vi "Balance Control Design.vi"() -> ()   [LabVIEW 2018]
uses:
  <vilib>/Analysis/baseanly.llb/Real A x B.vi
  <vilib>/Analysis/_algsub.llb/Real Matrix Rank.vi
  <vilib>/addons/Control Design/_Model Construction/Model Creation.llb/Model Creation SubVI/cd_Create State Space Model.vi
  <vilib>/addons/Control Design/_Model Construction/Model Information.llb/Model Information SubVIs/cd_Get Matrices From SS Model.vi
  <vilib>/Analysis/Matrix/Numeric/Subtract/Subtract - RM,RM.vi
  <vilib>/addons/Control Design/_Model Construction/Model Information.llb/Model Information SubVIs/cd_Set Matrices To SS Model.vi
  <vilib>/addons/Control Design/_Dynamic Analysis/Dynamic Analysis.llb/Dynamic Analysis subVI/cd_Pole-Zero Map (State-Space).vi
  <vilib>/addons/Control Design/_Model Construction/Model Information.llb/Model Information SubVIs/cd_Check State Space Model.vi
  <vilib>/Analysis/Matrix/Numeric/Conversions/Array To Matrix - RA2.vi
  <vilib>/Analysis/baseanly.llb/Real Inverse Matrix.vi
  <vilib>/addons/Control Design/_Utility/Model Viewer.llb/Model Viewer SubVI/cd_Draw State-Space Equation (SS).vi
  <vilib>/addons/Control Design/_Dynamic Analysis/NI_CD_Dynamic Analysis.lvlib
  <vilib>/addons/Control Design/_Model Construction/NI_LinSys_Model Creation.lvlib
  <vilib>/addons/Control Design/_Utility/NI_CD_Model Viewer.lvlib
  <vilib>/addons/Control Design/_State-Space Analysis/NI_CD_State-Space Analysis.lvlib
  <vilib>/Analysis/NI_AALPro.lvlib
  <vilib>/addons/Control Design/_Model Construction/NI_LinSys_Model Information.lvlib
  <vilib>/Analysis/NI_AALBase.lvlib
  <vilib>/Analysis/Matrix/NI_Matrix.lvlib
panel:
  out "K = Kc*W^(-1)":dbl[][](array[numeric])=[[-3.38528708742015, 41.477506482643726, -1.3825456536938336, 2.9377197211817103]] format="%#_3g"
  in  "Companion Gain: Kc":dbl[][](array[numeric])=[[19200.0, 7841.2, 1869.47, 75.59]] format="%#_5g"
  out "Closed Loop Poles":cdb[](array[numeric])=[-40.0087773566082+0.0i, -29.991275636401266+0.0i, -2.800173503495311+0.0i, -2.800173503495311+0.0i] format="%#_4g"
  out "Controllability: T":dbl[][](array[numeric])=[[0.0, 49.72, -0.517088, 7331.6752777152], [0.0, 49.13, -0.512116, 12848.9742260064], [49.72, -0.517088, 7331.6752777152, -152.67249356823805], [49.13, -0.512116, 12848.9742260064, -209.44995284046655]] format="%#_5g"
  out "W = T*Tc^(-1)":dbl[][](array[numeric])=[[-5671.601700000002, -3.6362146628449897e-16, 49.71999999999997, 0.0], [-4.279568108558251e-12, -0.0011640000000003648, 49.12999999999997, 0.0], [2.2428445845514195e-14, -5671.601700000003, 5.484558302927993e-16, 49.72], [-4.392598967657428e-14, -5.706092893409093e-12, -0.001163999999999423, 49.13]] format="%#_5g"
  out "Companion Form":picture
  out "Number of States":i32=4
  out "Controllable?":bool=TRUE
  out "Controllability Rank":i32=4
  out "Poles":cdb[](array[numeric])=[-16.174828889209856+0.0i, 16.168951670075447+0.0i, -0.004522780865591975+0.0i, 0.0+0.0i] caption="Open Loop Poles" format="%#_3g"
  out "Open Loop State-Space Model":picture
  in  "stop":bool
  # "Engineering Trainer Boards"
  # "Controls Board"
  # "Balance Control Design"
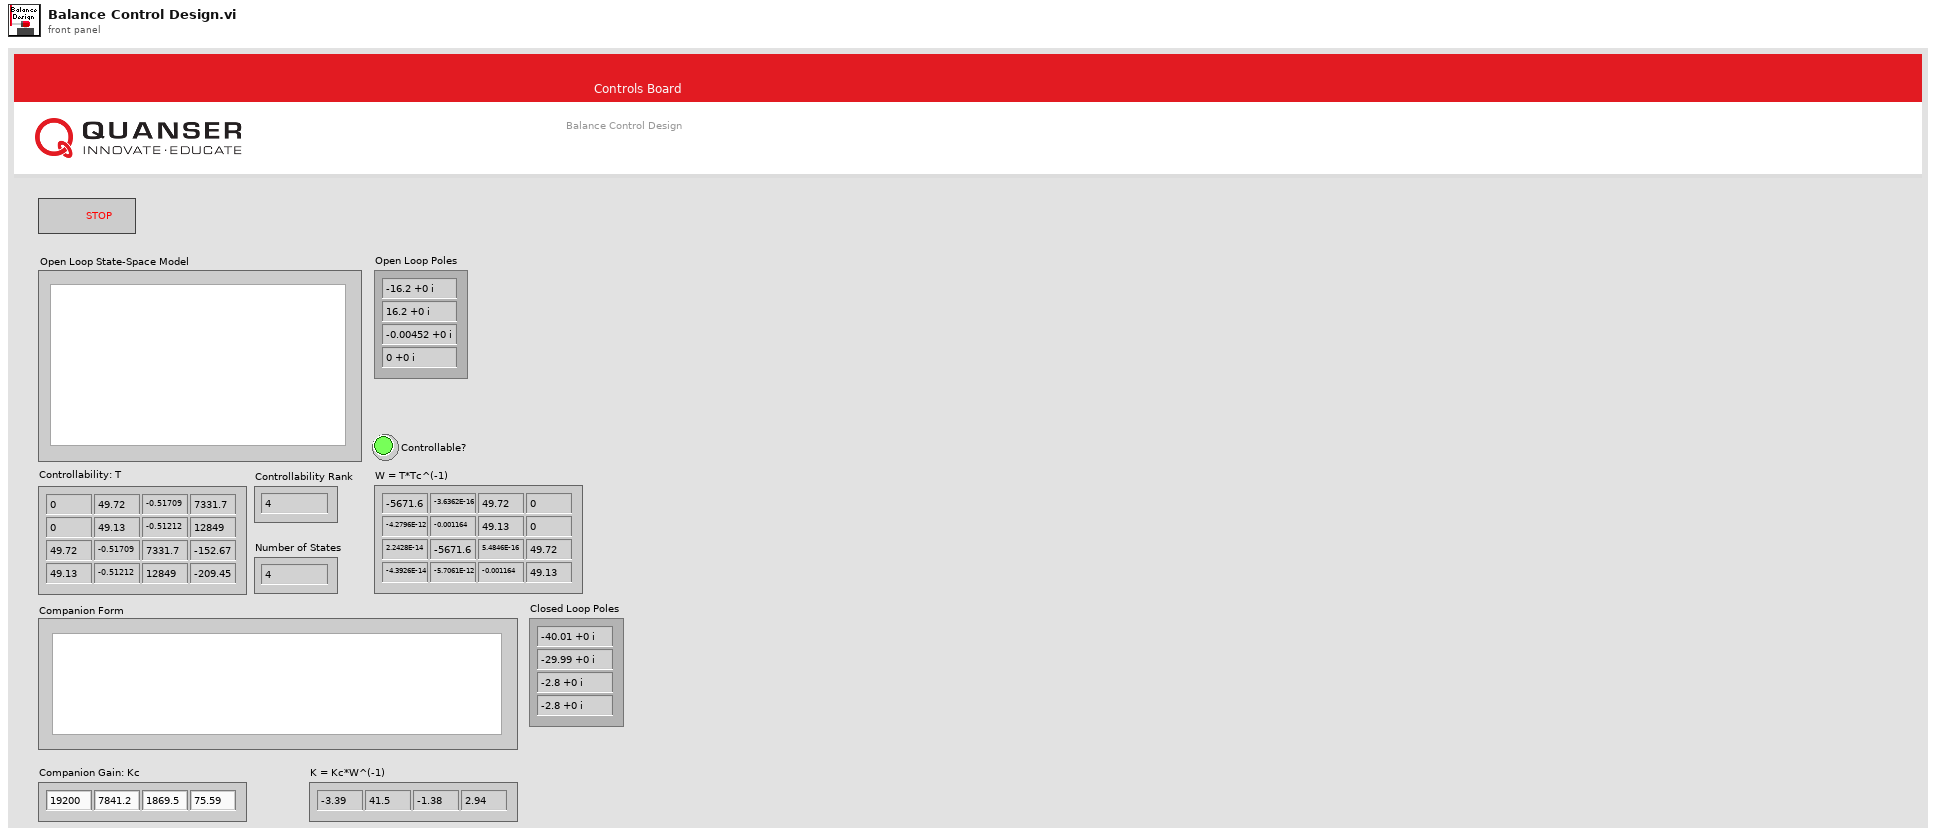
[diagram p1: front panel]
types:
  T1 = typedef "NI_LinSys_Model Typedefs.lvlib/CD State Space Model (MIMO).ctl" = cluster{"properties":T2, "A":dbl[][], "B":dbl[][], "C":dbl[][], "D":dbl[][], "StateNames":string[], "Transport Delay":dbl[][]}
  T2 = typedef "NI_LinSys_Model Typedefs.lvlib/CD General Elements.ctl" = cluster{"Model name":string, "Input names":string[], "Output names":string[], "Input Delays":dbl[], "Output Delays":dbl[], "Sampling Time":dbl, "Notes":string}
  T3 = typedef "NI_Matrix.lvlib/RealMatrix.ctl" = dbl[][]
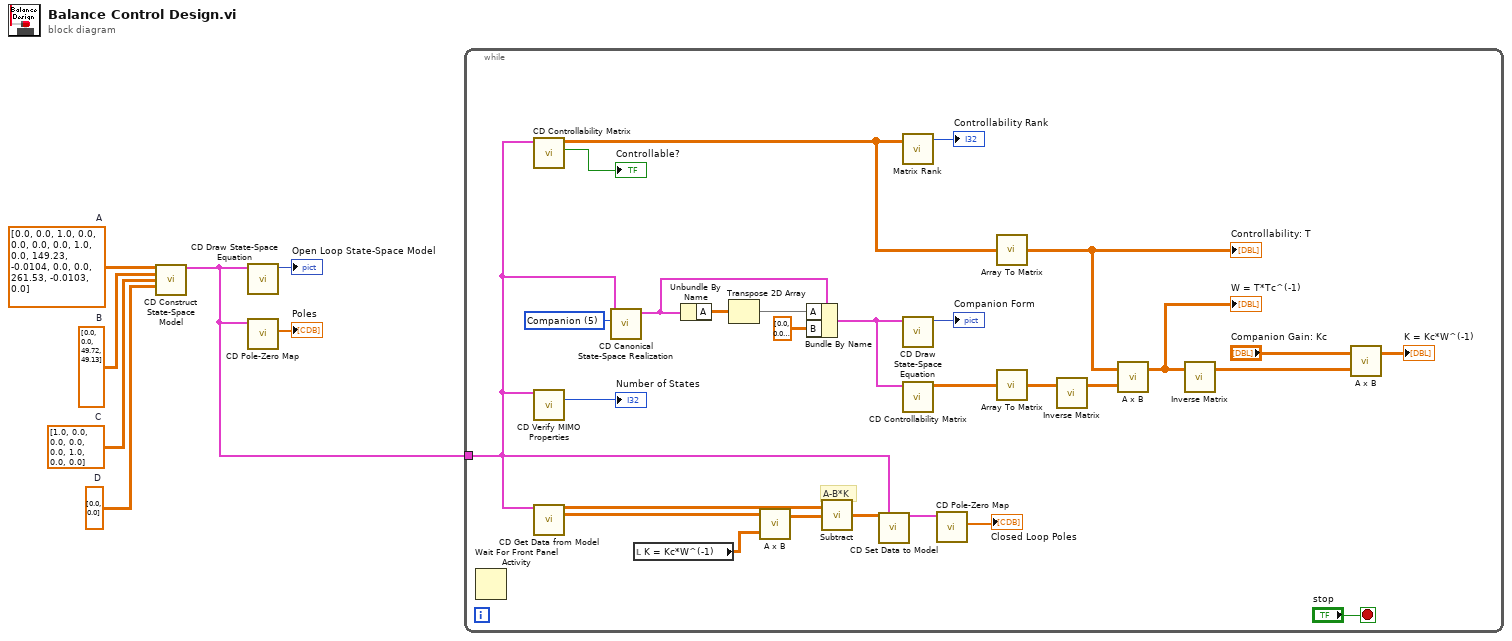
[diagram p0: block diagram]
diagram:
  w3 = dbl[][] [[0.0], [0.0]]  # D
  w4 = dbl[][] [[1.0, 0.0, 0.0, 0.0], [0.0, 1.0, 0.0, 0.0]]  # C
  w5 = dbl[][] [[0.0], [0.0], [49.72], [49.13]]  # B
  w6 = dbl[][] [[0.0, 0.0, 1.0, 0.0], [0.0, 0.0, 0.0, 1.0], [0.0, 149.23, -0.0104, 0.0], [0.0, 261.53, -0.0103, 0.0]]  # A
  n1 = call-poly <vilib>:"CD Construct State-Space Model.vi"("A"=w6, "B"=w5, "C"=w4, "D"=w3) -> ("State-Space Model"=w1:T1)  [unwired: 10 in, 1 out]
  n2 = call-poly <vilib>:"CD Draw State-Space Equation.vi"("State-Space Model"=w1) -> ("Equation"=→"Open Loop State-Space Model":picture)  [unwired: 8 in, 2 out]
  n3 = call-poly <vilib>:"CD Pole-Zero Map.vi"("State-Space Model"=w1) -> ("Poles"=→"Poles":cdb[])  [unwired: 7 in, 3 out]
  n4 = while {
    tunnel: w1 -> [w9]
    stop <- "stop" stop-if-true
    w14 = u16 5 items=["Modal"=0, "Companion"=5, "Controllability"=1, "Controller Companion"=2, "Observability"=3, "Observer Companion"=4] ("Form Type")
    # "A-B*K"
    n5 = Wait For Front Panel Activity() -> ()  [unwired: 3 in, 1 out]
    n6 = call <vilib>:"CD Controllability Matrix.vi"("State-Space Model"=w9) -> ("Is Controllable?"=→"Controllable?":bool, "Controllability Matrix"=w12:dbl[][])  [unwired: 7 in, 2 out]
    n7 = call-poly <vilib>:"CD Verify MIMO Properties.vi"("State-Space Model In"=w9) -> ("Number of States"=→"Number of States":i32)  [unwired: 9 in, 5 out]
    n8 = call-poly <vilib>:"CD Get Data from Model.vi"("State-Space Model"=w9) -> ("Matrix A"=w16:dbl[][], "Matrix B"=w17:dbl[][])  [unwired: 10 in, 3 out]
    n9 = call <vilib>:"CD Canonical State-Space Realization.vi"("Form Type"=w14, "State-Space Model"=w9) -> ("Transformed Model"=w29:T1)  [unwired: 7 in, 2 out]
    n10 = local read "K = Kc*W^(-1)"() -> (w19:dbl[][])
    n11 = Unbundle By Name(w29) -> ("A"=w31:dbl[][])
    n12 = Transpose 2D Array(2D array=w31) -> (transposed array=w28:dbl[][])
    n13 = call-poly <vilib>:"A x B.vi"("B"=w19, "A"=w17) -> ("A x B"=w13:T3)  [unwired: 1 out]
    n14 = Bundle By Name(cluster=w29, "A"=w28, "B"=dbl[][] [[0.0], [0.0], [0.0], [1.0]]) -> (w26:T1)
    n15 = call-poly <vilib>:"Subtract.vi"("Real Matrix B"=w13, "Real Matrix A"=w16) -> ("A - B"=w15:T3)
    n16 = call-poly <vilib>:"CD Set Data to Model.vi"("Matrix A"=w15, "State-Space Model In"=w9) -> ("Model Out"=w18:T1)  [unwired: 12 in, 1 out]
    n17 = call-poly <vilib>:"Matrix Rank.vi"("Input Matrix"=w12) -> ("rank"=→"Controllability Rank":i32)  [unwired: 1 in, 1 out]
    n18 = call-poly <vilib>:"CD Draw State-Space Equation.vi"("State-Space Model"=w26) -> ("Equation"=→"Companion Form":picture)  [unwired: 8 in, 2 out]
    n19 = call <vilib>:"CD Controllability Matrix.vi"("State-Space Model"=w26) -> ("Controllability Matrix"=w25:dbl[][])  [unwired: 7 in, 3 out]
    n20 = call-poly <vilib>:"CD Pole-Zero Map.vi"("State-Space Model"=w18) -> ("Poles"=→"Closed Loop Poles":cdb[])  [unwired: 7 in, 3 out]
    n21 = call-poly <vilib>:"Array To Matrix.vi"("Real 2D Array"=w12) -> ("Real Matrix"=w22:T3)
    "Controllability: T" <- w22
    n22 = call-poly <vilib>:"Array To Matrix.vi"("Real 2D Array"=w25) -> ("Real Matrix"=w24:T3)
    n23 = call-poly <vilib>:"Inverse Matrix.vi"("Input Matrix"=w24) -> ("Inverse Matrix"=w23:T3)  [unwired: 1 in, 1 out]
    n24 = call-poly <vilib>:"A x B.vi"("B"=w23, "A"=w22) -> ("A x B"=w21:T3)  [unwired: 1 out]
    "W = T*Tc^(-1)" <- w21
    n25 = call-poly <vilib>:"Inverse Matrix.vi"("Input Matrix"=w21) -> ("Inverse Matrix"=w20:T3)  [unwired: 1 in, 1 out]
    n26 = call-poly <vilib>:"A x B.vi"("B"=w20, "A"="Companion Gain: Kc") -> ("A x B"=→"K = Kc*W^(-1)":T3)  [unwired: 1 out]
  }
